vi "update-graphlegendOD.vi"(0 "XYGraph in":refnum<vi>, 1 "plot names":string[](array[string])=["part", "full"]) -> ()   [LabVIEW 2015]
panel:
  out "error out":errorcluster
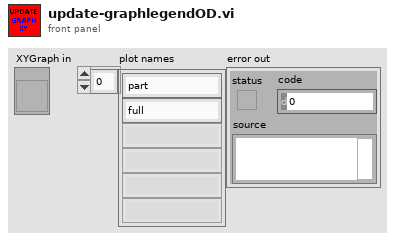
[diagram p1: front panel]
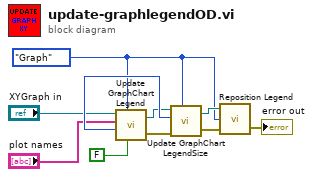
[diagram p0: block diagram]
diagram:
  w2 = enum16{"Chart", "Graph"}."Graph" ("Display Type")
  n1 = call "Update GraphChart Legend.vi"("Legend:Autosize"=FALSE, "Display Type"=w2, "Plot Names"="plot names", "GraphChart Reference in"="XYGraph in") -> ("error out"=w10:errorcluster, "GraphChart Reference out"=w4:refnum<vi>, "# Plots"=w9:i32)  [unwired: 1 in]
  n2 = call "Update GraphChart LegendSize.vi"("GraphChart Reference"=w4, "# Plots"=w9, "error in (no error)"=w10, "Display Type"=w2) -> ("GraphChart Reference out"=w3:refnum<vi>, "error out"=w8:errorcluster)  [unwired: 1 in]
  n3 = call "Reposition Legend.vi"("error in (no error)"=w8, "Display Type"=w2, "GraphChart in"=w3) -> ("error out"=→"error out":errorcluster)  [unwired: 1 out]
